vi "Write Save Image.lvclass.vi"(8 "error in (no error)":errorcluster, 10 "Save Image.lvclass":refnum<class "Save Image.lvclass">, 11 "Image Constructor in":refnum<class "Image Constructor.lvclass">) -> (0 "error out":errorcluster, 3 "Image Constructor out":refnum<class "Image Constructor.lvclass">)   [LabVIEW 2018]
uses:
  Image Constructor.lvclass
  C:/Users/observer/Desktop/SPARC4_ACS/Simulated_Image_Constructor/Simulated_Image_Constructor.lvclass
  Save Image/Save Image.lvclass
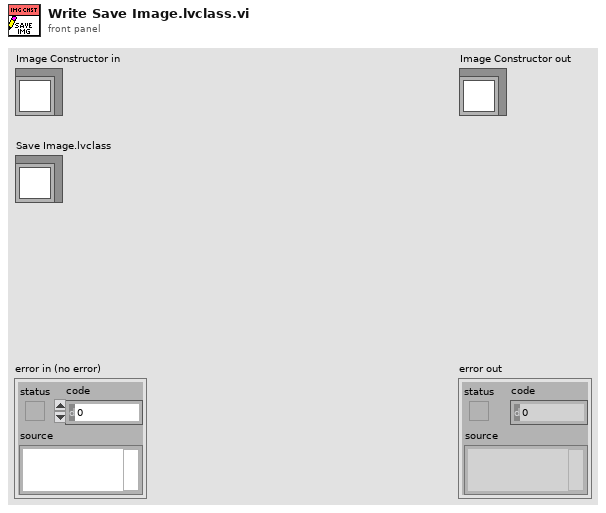
[diagram p1: front panel]
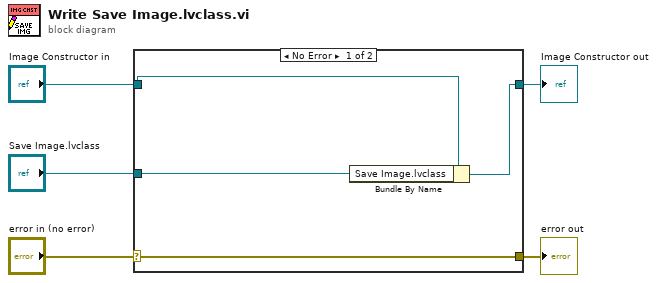
[diagram p0: block diagram]
diagram:
  n1 = case shown="No Error" "error in (no error)" {
    selector: "error in (no error)" -> [w9 w10]
    tunnel: [w9 w10] -> w4
    tunnel: [w7 w11] -> w2
    tunnel: "Image Constructor in" -> [w8 w11]
    tunnel: "Save Image.lvclass" -> [w6 _]
    frame No Error {
      n2 = Bundle By Name(cluster=w8, "Save Image.lvclass"=w6) -> (w7:refnum<class "Image Constructor.lvclass">)
    }
    frame Error {
    }
  }
  "error out" <- w4
  "Image Constructor out" <- w2
